vi "Save Image.vi"(8 "error in (no error)":errorcluster, 11 "IMAQ Display in":refnum<class "HIJ IMAQdx Display.lvclass">) -> (0 "error out":errorcluster, 3 "IMAQ Display out":refnum<class "HIJ IMAQdx Display.lvclass">)   [LabVIEW 2014, in "HIJ IMAQdx Display.lvlib" / "HIJ IMAQdx Display.lvclass"]
doc: "Speichert das Kamerabild in PNG Format und ruft Generate Report auf. Wenn Flag \"Time in Filename\" gesetzt ist, wird ein Zeitstempel dem Dateinamen angehängt."
uses:
  HIJ IMAQdx Display.lvclass
  HIJ IMAQdx Display.lvclass/HIJ IMAQdx Display.ctl
  HIJ Vision Display/HIJ Vision Display/HIJ Vision Display.lvclass/HIJ Vision Display.ctl
  HIJ Vision Display/HIJ Vision Display/Read Display Image 2.vi
  HIJ Vision Display/HIJ Vision Display/Read WorkDir.vi
  HIJ Vision Display/HIJ Vision Display/Read Image Source Name.vi
  <vilib>/Utility/config.llb/NI_LVConfig.lvlib
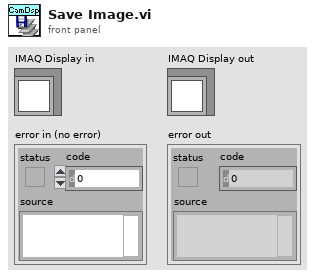
[diagram p1: front panel]
types:
  T1 = typedef "IMAQ Image.ctl" = refnum<image>
  T2 = typedef "NI_LVConfig.lvlib/Config Data RefNum.ctl" = refnum<k1>
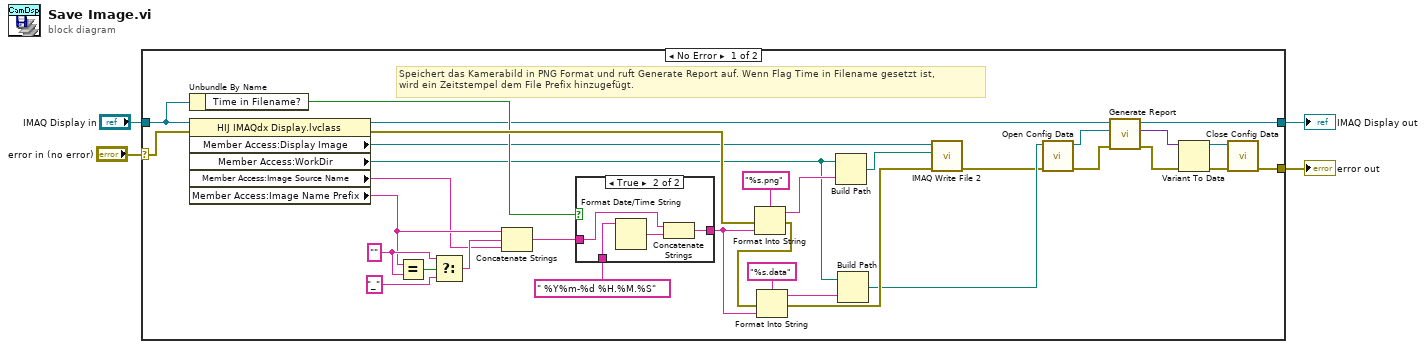
[diagram p0: block diagram]
diagram:
  n1 = case shown="No Error" "error in (no error)" {
    selector: "error in (no error)" -> [w22 w44]
    tunnel: [w6 w44] -> w3
    tunnel: [w11 w43] -> w1
    tunnel: "IMAQ Display in" -> [w27 w43]
    frame No Error {
      w29 = "" ("y")
      # "Speichert das Kamerabild in PNG Format und ruft Generate Report auf. Wenn Flag Time in Filename gesetzt ist, \nwird ein Zeitstempel dem File Prefix hinzugefügt."
      n2 = Unbundle By Name(w27) -> ("Time in Filename?"=w35:bool)
      n3 = property class="HIJ IMAQdx Display.lvclass"(reference=w27, error in=w22) -> (reference out=w23:refnum<class "HIJ IMAQdx Display.lvclass">, error out=w36:errorcluster, "Member Access:Display Image"=w26:T1, "Member Access:WorkDir"=w16:path, "Member Access:Image Source Name"=w24:string, "Member Access:Image Name Prefix"=w25:string)
      n4 = Equal?(x=w25, y=w29) -> (x = y?=w31:bool)
      n5 = Select(t=w29, s=w31, f="_" ("string")) -> (s? t:f=w30:string)
      n6 = Concatenate Strings(w25, w30, w24) -> (w34:string)
      n7 = case shown="True" w35 {
        tunnel: [w38 w40] -> w17
        tunnel: w34 -> [w38 w39]
        tunnel: " %Y%m-%d %H.%M.%S" ("time format string (%c)") -> [_ w42]
        frame False {
        }
        frame True {
          n8 = Format Date/Time String(time format string (%c)=w42) -> (date/time string=w41:string)  [unwired: 2 in]
          n9 = Concatenate Strings(w39, w41) -> (w40:string)
        }
      }
      n10 = Format Into String(format string="%s.png", error in=w36, w17) -> (resulting string=w20:string, error out=w5:errorcluster)  [unwired: 1 in]
      n11 = Format Into String(format string="%s.data", error in=w5, w17) -> (resulting string=w15:string, error out=w37:errorcluster)  [unwired: 1 in]
      n12 = Build Path(base path=w16, name or relative path=w20) -> (appended path=w32:path)
      n13 = Build Path(base path=w16, name or relative path=w15) -> (appended path=w19:path)
      n14 = call-poly "IMAQ Write File 2"("error in (no error)"=w37, "File Path"=w32, "Image"=w26) -> ("error out"=w14:errorcluster)  [unwired: 7 in, 1 out]
      n15 = call <vilib>:"Open Config Data.vi"("error in (no error)"=w14, "configuration file path"=w19) -> ("error out"=w13:errorcluster, "refnum"=w12:T2)  [unwired: 7 in, 1 out]
      n16 = call-dynamic "Generate Report.vi"("error in (no error)"=w13, "Resource In"=w12, "HIJ IMAQdx Display in"=w23) -> ("error out"=w10:errorcluster, "Resource Out"=w8:variant, "HIJ IMAQdx Display out"=w11:refnum<class "HIJ IMAQdx Display.lvclass">)  [unwired: 6 in]
      n17 = Variant To Data(error in=w10, Variant=w8) -> (data=w7:T2, error out=w9:errorcluster)  [unwired: 1 in]
      n18 = call <vilib>:"Close Config Data.vi"("error in (no error)"=w9, "refnum"=w7) -> ("error out"=w6:errorcluster)  [unwired: 8 in, 1 out]
    }
    frame Error {
    }
  }
  "error out" <- w3
  "IMAQ Display out" <- w1
